vi "Create CONNECT Packet (5.0).vi"(5 "type":refnum<class "CONNECT.lvclass">, 6 "Keep Alive (s)":u16, 7 "Client ID (empty: generate new)":string, 8 "error in (no error)":errorcluster, 10 "Payload":T1, 11 "Connect Flags":T2) -> (0 "error out":errorcluster, 2 "Bytes Stream":u8[](array[numeric]) format="%08b", 3 "CONNECT":refnum<class "CONNECT.lvclass">)   [LabVIEW 2013, in "MQTT_Control_Packets_50.lvlib" / "CONNECT_50.lvclass"]
uses:
  CONNECT_50.lvclass
  CONNECT/CONNECT.lvclass
  ConnectFlags (v5.0) -- cluster.ctl
  CONNECT/ConnectPayload -- cluster.ctl
  ControlPacket/ControlPacket.lvclass/ControlPacket.ctl
  ControlPacket/ControlPacket.lvclass
  MQTT_50/MQTTVersion50.lvclass
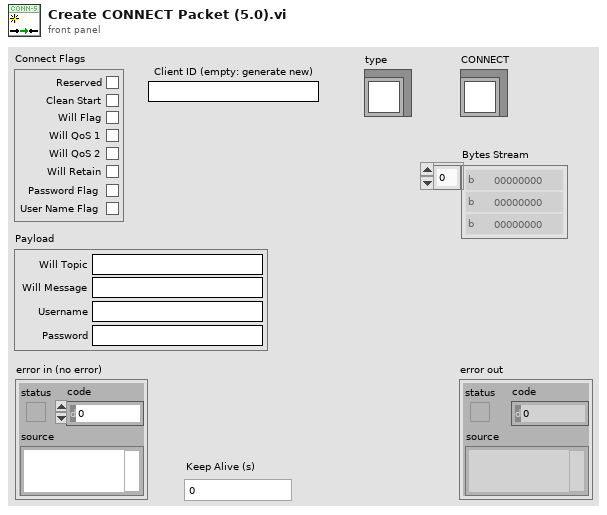
[diagram p1: front panel]
types:
  T1 = typedef "MQTT_Control_Packets.lvlib/CONNECT.lvclass/ConnectPayload -- cluster.ctl" = cluster{"Will Topic":string, "Will Message":string, "Username":string, "Password":string}
  T2 = typedef "MQTT_Control_Packets_50.lvlib/CONNECT_50.lvclass/ConnectFlags (v5.0) -- cluster.ctl" = cluster{"Reserved":bool, "Clean Start":bool, "Will Flag":bool, "Will QoS 1":bool, "Will QoS 2":bool, "Will Retain":bool, "Password Flag":bool, "User Name Flag":bool}
  T3 = typedef "MQTT_Control_Packets.lvlib/CONNECT.lvclass/ConnectFlags -- cluster.ctl" = cluster{"Reserved":bool, "Clean Session":bool, "Will Flag":bool, "Will QoS 1":bool, "Will QoS 2":bool, "Will Retain":bool, "Password Flag":bool, "User Name Flag":bool}
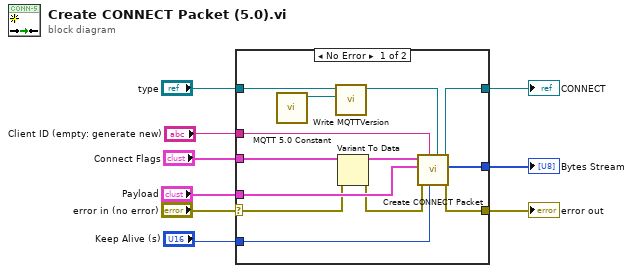
[diagram p0: block diagram]
diagram:
  n1 = case shown="No Error" "error in (no error)" {
    selector: "error in (no error)" -> [w11 w24]
    tunnel: [w15 w24] -> w8
    tunnel: [w19 w23] -> w7
    tunnel: "Connect Flags" -> [w13 _]
    tunnel: "Keep Alive (s)" -> [w17 _]
    tunnel: "Client ID (empty: generate new)" -> [w16 _]
    tunnel: "Payload" -> [w18 _]
    tunnel: [w14 _] -> w2
    tunnel: "type" -> [w21 w23]
    frame No Error {
      n2 = call "MQTT 5.0 Constant.vi"() -> ("MQTT 5.0 Constant"=w22:refnum<class "MQTTVersion50.lvclass">)  [unwired: 11 in]
      n3 = call "Write MQTTVersion.vi"("MQTTVersion"=w22, "ControlPacket in"=w21) -> ("ControlPacket out"=w20:refnum<class "CONNECT.lvclass">)  [unwired: 9 in]
      n4 = Variant To Data(error in=w11, Variant=w13) -> (data=w12:T3, error out=w10:errorcluster)  [unwired: 1 in]
      n5 = call "Create CONNECT Packet.vi"("type"=w20, "Keep Alive (s)"=w17, "Client ID (empty: generate new)"=w16, "error in (no error)"=w10, "Payload"=w18, "Connect Flags"=w12) -> ("error out"=w15:errorcluster, "Bytes Stream"=w14:u8[], "CONNECT"=w19:refnum<class "CONNECT.lvclass">)  [unwired: 3 in]
    }
    frame Error {
    }
  }
  "error out" <- w8
  "CONNECT" <- w7
  "Bytes Stream" <- w2
